vi "Acquire.vi"(8 "error in (no error)":errorcluster, 9 "Initialize":bool, 10 "Reply to":refnum<class "Result Reply Msg.lvclass">, 11 "Pulse Recorder in":refnum<class "Pulse Recorder.lvclass">) -> (0 "error out":errorcluster, 3 "Pulse Recorder out":refnum<class "Pulse Recorder.lvclass">)   [LabVIEW 2015, in "Pulse Recorder.lvclass"]
uses:
  Pulse Recorder.lvclass
  Measure Object Messages/Result Reply Msg/Result Reply Msg.lvclass
  Measure Object/Measure Object.lvclass
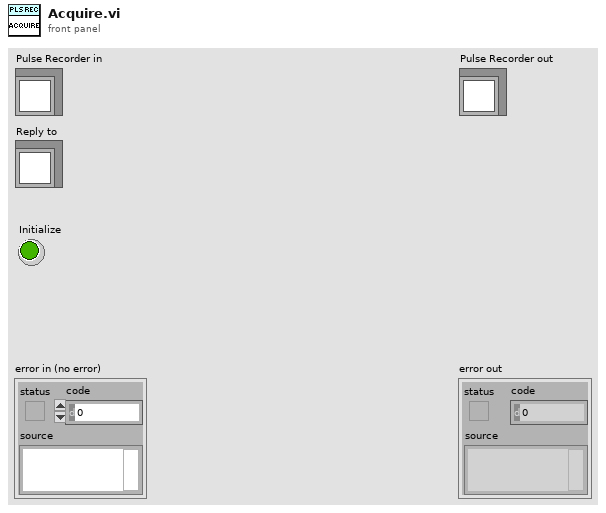
[diagram p1: front panel]
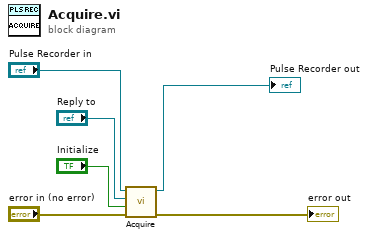
[diagram p0: block diagram]
diagram:
  n1 = call-parent "Acquire.vi"("error in (no error)"="error in (no error)", "Initialize"="Initialize", "Reply to"="Reply to", "Measure Object in"="Pulse Recorder in") -> ("error out"=→"error out":errorcluster, "Measure Object out"=→"Pulse Recorder out":refnum<class "Pulse Recorder.lvclass">)  [unwired: 6 in]
